vi "ConvertLVClustertoFGNetFDMString.vi"(1 "Cluster":T1={"Version"={"version"=20, "pad"=0}, "Positions"={"Doubles"={"longitude"=0.0, "latitude"=0.0, "altitude"=0.0}, "Singles"={"agl"=0.0, "phi"=0.0, "theta"=0.0, "psi"=0.0, "alpha"=0.0, "beta"=0.0}}, "Velocities"={"phidot"=0.0, "thetadot"=0.0, "psidot"=0.0, "vcas"=0.0, "climb_rate"=0.0, "v_north"=0.0, "v_east"=0.0, "v_down"=0.0, "v_wind_body_north"=0.0, "v_wind_body_east"=0.0, "v_wind_body_down"=0.0}, "Accelerations"={"A_X_pilot"=0.0, "A_Y_pilot"=0.0, "A_Z_pilot"=0.0}, "Stall"={"stall_warning"=0.0, "slip_deg"=0.0}, "Engine Status"={"num_engines"=0, "eng_state"=[0, 0, 0, 0], "rpm"=[0.0, 0.0, 0.0, 0.0], "fuel_flow"=[0.0, 0.0, 0.0, 0.0], "fuel_px"=[0.0, 0.0, 0.0, 0.0], "egt"=[0.0, 0.0, 0.0, 0.0], "cht"=[0.0, 0.0, 0.0, 0.0], "mp_osi"=[0.0, 0.0, 0.0, 0.0], "tit"=[0.0, 0.0, 0.0, 0.0], "oil_temp"=[0.0, 0.0, 0.0, 0.0], "oil_px"=[0.0, 0.0, 0.0, 0.0]}, "Consumables"={"num_tanks"=0, "fuel_quantity"=[0.0, 0.0, 0.0, 0.0]}, "Gear Status"={"num_wheels"=0, "wow"=[0, 0, 0, 0], "gear_pos"=[0.0, 0.0, 0.0, 0.0], "gear_steer"=[0.0, 0.0, 0.0, 0.0], "gear_compression"=[0.0, 0.0, 0.0, 0.0]}, "Environment"={"curr_time"=0, "warp"=0, "visibility"=0.0}, "Control Surface Positions"={"elevator"=0.0, "elevator_trim_tab"=0.0, "left_flap"=0.0, "right_flap"=0.0, "left aileron"=0.0, "right_aileron"=0.0, "rudder"=0.0, "nose_wheel"=0.0, "speedbrake"=0.0, "spoilers"=0.0}}) -> (0 "FGNetFDM":string)   [LabVIEW 2010, in "Flight Gear Interface Custom Device.lvlib"]
uses:
  Flight Gear Interface Custom Device.lvlib
  FGNetFDM.ctl
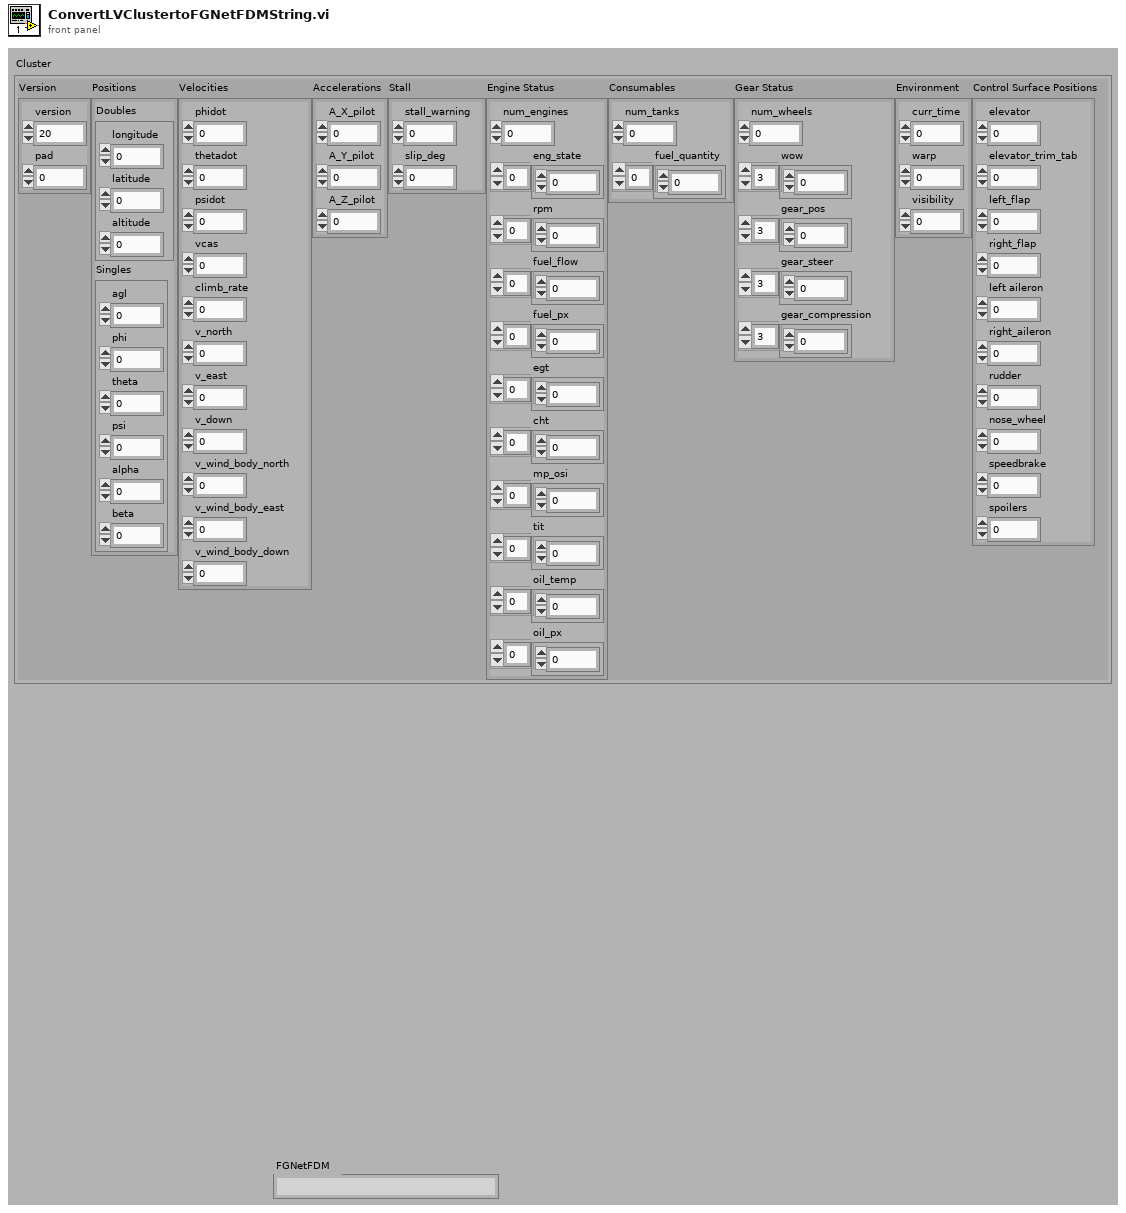
[diagram p1: front panel]
types:
  T1 = typedef "Flight Gear Interface Custom Device.lvlib/FGNetFDM.ctl" = cluster{"Version":cluster{"version":u32, "pad":u32}, "Positions":cluster{"Doubles":cluster{"longitude":dbl, "latitude":dbl, "altitude":dbl}, "Singles":cluster{"agl":sgl, "phi":sgl, "theta":sgl, "psi":sgl, "alpha":sgl, "beta":sgl}}, "Velocities":cluster{"phidot":sgl, "thetadot":sgl, "psidot":sgl, "vcas":sgl, "climb_rate":sgl, "v_north":sgl, "v_east":sgl, "v_down":sgl, "v_wind_body_north":sgl, "v_wind_body_east":sgl, "v_wind_body_down":sgl}, "Accelerations":cluster{"A_X_pilot":sgl, "A_Y_pilot":sgl, "A_Z_pilot":sgl}, "Stall":cluster{"stall_warning":sgl, "slip_deg":sgl}, "Engine Status":cluster{"num_engines":u32, "eng_state":u32[], "rpm":sgl[], "fuel_flow":sgl[], "fuel_px":sgl[], "egt":sgl[], "cht":sgl[], "mp_osi":sgl[], "tit":sgl[], "oil_temp":sgl[], "oil_px":sgl[]}, "Consumables":cluster{"num_tanks":u32, "fuel_quantity":sgl[]}, "Gear Status":cluster{"num_wheels":u32, "wow":u32[], "gear_pos":sgl[], "gear_steer":sgl[], "gear_compression":sgl[]}, "Environment":cluster{"curr_time":u32, "warp":i32, "visibility":sgl}, "Control Surface Positions":cluster{"elevator":sgl, "elevator_trim_tab":sgl, "left_flap":sgl, "right_flap":sgl, "left aileron":sgl, "right_aileron":sgl, "rudder":sgl, "nose_wheel":sgl, "speedbrake":sgl, "spoilers":sgl}}
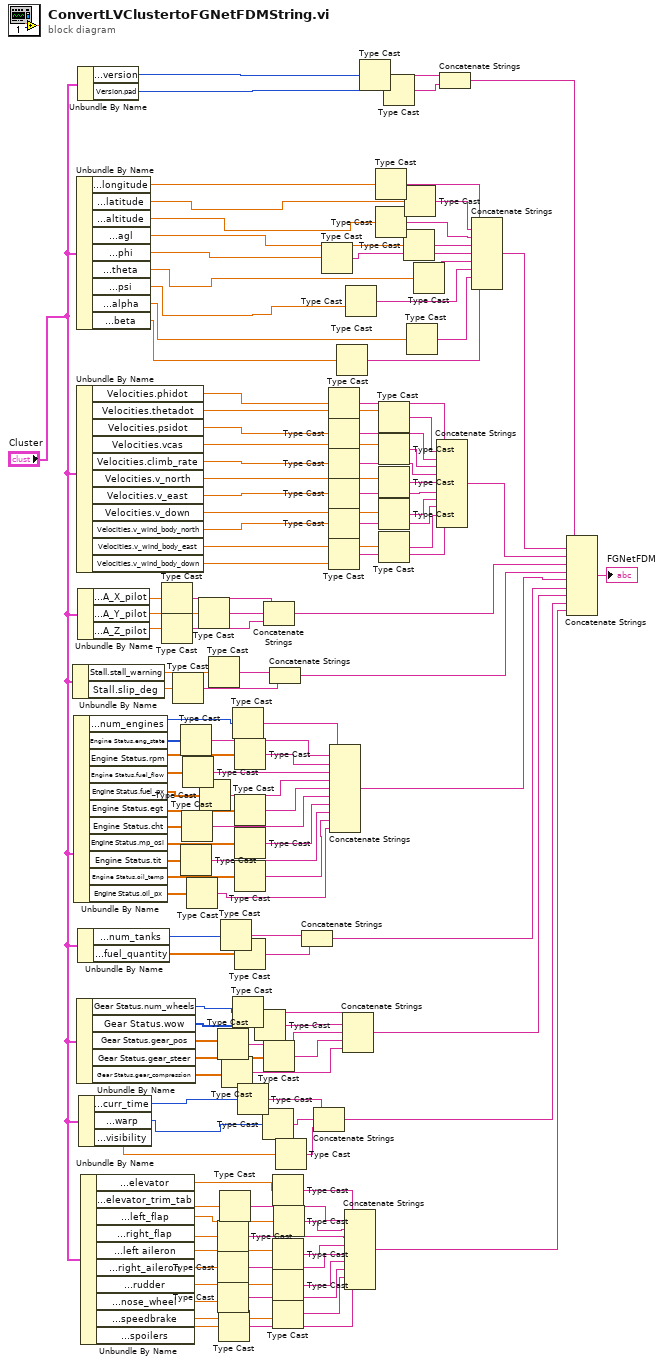
[diagram p0: block diagram]
diagram:
  n1 = Unbundle By Name("Cluster") -> ("Stall.stall_warning"=w100:sgl, "Stall.slip_deg"=w99:sgl)
  n2 = Unbundle By Name("Cluster") -> ("Engine Status.num_engines"=w7:u32, "Engine Status.eng_state"=w98:u32[], "Engine Status.rpm"=w97:sgl[], "Engine Status.fuel_flow"=w56:sgl[], "Engine Status.fuel_px"=w1:sgl[], "Engine Status.egt"=w96:sgl[], "Engine Status.cht"=w95:sgl[], "Engine Status.mp_osi"=w94:sgl[], "Engine Status.tit"=w93:sgl[], "Engine Status.oil_temp"=w92:sgl[], "Engine Status.oil_px"=w91:sgl[])
  n3 = Unbundle By Name("Cluster") -> ("Positions.Doubles.longitude"=w13:dbl, "Positions.Doubles.latitude"=w12:dbl, "Positions.Doubles.altitude"=w11:dbl, "Positions.Singles.agl"=w117:sgl, "Positions.Singles.phi"=w10:sgl, "Positions.Singles.theta"=w9:sgl, "Positions.Singles.psi"=w8:sgl, "Positions.Singles.alpha"=w116:sgl, "Positions.Singles.beta"=w115:sgl)
  n4 = Unbundle By Name("Cluster") -> ("Velocities.phidot"=w114:sgl, "Velocities.thetadot"=w108:sgl, "Velocities.psidot"=w113:sgl, "Velocities.vcas"=w107:sgl, "Velocities.climb_rate"=w112:sgl, "Velocities.v_north"=w106:sgl, "Velocities.v_east"=w111:sgl, "Velocities.v_down"=w105:sgl, "Velocities.v_wind_body_north"=w110:sgl, "Velocities.v_wind_body_east"=w104:sgl, "Velocities.v_wind_body_down"=w109:sgl)
  n5 = Unbundle By Name("Cluster") -> ("Gear Status.num_wheels"=w5:u32, "Gear Status.wow"=w89:u32[], "Gear Status.gear_pos"=w88:sgl[], "Gear Status.gear_steer"=w87:sgl[], "Gear Status.gear_compression"=w86:sgl[])
  n6 = Unbundle By Name("Cluster") -> ("Version.version"=w16:u32, "Version.pad"=w128:u32)
  n7 = Unbundle By Name("Cluster") -> ("Accelerations.A_X_pilot"=w103:sgl, "Accelerations.A_Y_pilot"=w102:sgl, "Accelerations.A_Z_pilot"=w101:sgl)
  n8 = Unbundle By Name("Cluster") -> ("Consumables.num_tanks"=w6:u32, "Consumables.fuel_quantity"=w90:sgl[])
  n9 = Unbundle By Name("Cluster") -> ("Environment.curr_time"=w15:u32, "Environment.warp"=w14:i32, "Environment.visibility"=w17:sgl)
  n10 = Unbundle By Name("Cluster") -> ("Control Surface Positions.elevator"=w85:sgl, "Control Surface Positions.elevator_trim_tab"=w84:sgl, "Control Surface Positions.left_flap"=w83:sgl, "Control Surface Positions.right_flap"=w82:sgl, "Control Surface Positions.left aileron"=w81:sgl, "Control Surface Positions.right_aileron"=w80:sgl, "Control Surface Positions.rudder"=w79:sgl, "Control Surface Positions.nose_wheel"=w78:sgl, "Control Surface Positions.speedbrake"=w77:sgl, "Control Surface Positions.spoilers"=w76:sgl)
  n11 = Type Cast(x=w103) -> (*(type *) &x=w64:string)  [unwired: 1 in]
  n12 = Type Cast(x=w101) -> (*(type *) &x=w62:string)  [unwired: 1 in]
  n13 = Type Cast(x=w99) -> (*(type *) &x=w60:string)  [unwired: 1 in]
  n14 = Type Cast(x=w98) -> (*(type *) &x=w58:string)  [unwired: 1 in]
  n15 = Type Cast(x=w93) -> (*(type *) &x=w52:string)  [unwired: 1 in]
  n16 = Type Cast(x=w95) -> (*(type *) &x=w54:string)  [unwired: 1 in]
  n17 = Type Cast(x=w56) -> (*(type *) &x=w55:string)  [unwired: 1 in]
  n18 = Type Cast(x=w91) -> (*(type *) &x=w50:string)  [unwired: 1 in]
  n19 = Type Cast(x=w102) -> (*(type *) &x=w63:string)  [unwired: 1 in]
  n20 = Type Cast(x=w1) -> (*(type *) &x=w2:string)  [unwired: 1 in]
  n21 = Type Cast(x=w100) -> (*(type *) &x=w61:string)  [unwired: 1 in]
  n22 = Type Cast(x=w88) -> (*(type *) &x=w19:string)  [unwired: 1 in]
  n23 = Type Cast(x=w82) -> (*(type *) &x=w37:string)  [unwired: 1 in]
  n24 = Type Cast(x=w80) -> (*(type *) &x=w35:string)  [unwired: 1 in]
  n25 = Type Cast(x=w78) -> (*(type *) &x=w33:string)  [unwired: 1 in]
  n26 = Type Cast(x=w76) -> (*(type *) &x=w31:string)  [unwired: 1 in]
  n27 = Type Cast(x=w84) -> (*(type *) &x=w39:string)  [unwired: 1 in]
  n28 = Type Cast(x=w6) -> (*(type *) &x=w49:string)  [unwired: 1 in]
  n29 = Type Cast(x=w86) -> (*(type *) &x=w44:string)  [unwired: 1 in]
  n30 = Type Cast(x=w7) -> (*(type *) &x=w59:string)  [unwired: 1 in]
  n31 = Type Cast(x=w5) -> (*(type *) &x=w47:string)  [unwired: 1 in]
  n32 = Type Cast(x=w97) -> (*(type *) &x=w57:string)  [unwired: 1 in]
  n33 = Type Cast(x=w96) -> (*(type *) &x=w3:string)  [unwired: 1 in]
  n34 = Type Cast(x=w94) -> (*(type *) &x=w53:string)  [unwired: 1 in]
  n35 = Type Cast(x=w92) -> (*(type *) &x=w51:string)  [unwired: 1 in]
  n36 = Type Cast(x=w90) -> (*(type *) &x=w48:string)  [unwired: 1 in]
  n37 = Type Cast(x=w15) -> (*(type *) &x=w43:string)  [unwired: 1 in]
  n38 = Type Cast(x=w89) -> (*(type *) &x=w46:string)  [unwired: 1 in]
  n39 = Type Cast(x=w14) -> (*(type *) &x=w42:string)  [unwired: 1 in]
  n40 = Concatenate Strings(w64, w63, w62) -> (w27:string)
  n41 = Type Cast(x=w87) -> (*(type *) &x=w45:string)  [unwired: 1 in]
  n42 = Concatenate Strings(w61, w60) -> (w26:string)
  n43 = Type Cast(x=w85) -> (*(type *) &x=w40:string)  [unwired: 1 in]
  n44 = Type Cast(x=w81) -> (*(type *) &x=w36:string)  [unwired: 1 in]
  n45 = Type Cast(x=w79) -> (*(type *) &x=w34:string)  [unwired: 1 in]
  n46 = Type Cast(x=w77) -> (*(type *) &x=w32:string)  [unwired: 1 in]
  n47 = Type Cast(x=w83) -> (*(type *) &x=w38:string)  [unwired: 1 in]
  n48 = Type Cast(x=w17) -> (*(type *) &x=w41:string)  [unwired: 1 in]
  n49 = Concatenate Strings(w49, w48) -> (w24:string)
  n50 = Concatenate Strings(w43, w42, w41) -> (w22:string)
  n51 = Type Cast(x=w10) -> (*(type *) &x=w122:string)  [unwired: 1 in]
  n52 = Type Cast(x=w114) -> (*(type *) &x=w75:string)  [unwired: 1 in]
  n53 = Type Cast(x=w113) -> (*(type *) &x=w73:string)  [unwired: 1 in]
  n54 = Type Cast(x=w112) -> (*(type *) &x=w71:string)  [unwired: 1 in]
  n55 = Type Cast(x=w111) -> (*(type *) &x=w69:string)  [unwired: 1 in]
  n56 = Type Cast(x=w110) -> (*(type *) &x=w67:string)  [unwired: 1 in]
  n57 = Type Cast(x=w109) -> (*(type *) &x=w65:string)  [unwired: 1 in]
  n58 = Concatenate Strings(w59, w58, w57, w55, w2, w3, w54, w53, w52, w51, w50) -> (w25:string)
  n59 = Type Cast(x=w115) -> (*(type *) &x=w118:string)  [unwired: 1 in]
  n60 = Concatenate Strings(w47, w46, w19, w45, w44) -> (w23:string)
  n61 = Concatenate Strings(w40, w39, w38, w37, w36, w35, w34, w33, w32, w31) -> (w21:string)
  n62 = Type Cast(x=w8) -> (*(type *) &x=w120:string)  [unwired: 1 in]
  n63 = Type Cast(x=w16) -> (*(type *) &x=w18:string)  [unwired: 1 in]
  n64 = Type Cast(x=w13) -> (*(type *) &x=w126:string)  [unwired: 1 in]
  n65 = Type Cast(x=w11) -> (*(type *) &x=w124:string)  [unwired: 1 in]
  n66 = Type Cast(x=w108) -> (*(type *) &x=w74:string)  [unwired: 1 in]
  n67 = Type Cast(x=w107) -> (*(type *) &x=w72:string)  [unwired: 1 in]
  n68 = Type Cast(x=w106) -> (*(type *) &x=w70:string)  [unwired: 1 in]
  n69 = Type Cast(x=w105) -> (*(type *) &x=w68:string)  [unwired: 1 in]
  n70 = Type Cast(x=w104) -> (*(type *) &x=w66:string)  [unwired: 1 in]
  n71 = Type Cast(x=w128) -> (*(type *) &x=w127:string)  [unwired: 1 in]
  n72 = Type Cast(x=w117) -> (*(type *) &x=w123:string)  [unwired: 1 in]
  n73 = Type Cast(x=w12) -> (*(type *) &x=w125:string)  [unwired: 1 in]
  n74 = Type Cast(x=w116) -> (*(type *) &x=w119:string)  [unwired: 1 in]
  n75 = Type Cast(x=w9) -> (*(type *) &x=w121:string)  [unwired: 1 in]
  n76 = Concatenate Strings(w75, w74, w73, w72, w71, w70, w69, w68, w67, w66, w65) -> (w28:string)
  n77 = Concatenate Strings(w18, w127) -> (w30:string)
  n78 = Concatenate Strings(w126, w125, w124, w123, w122, w121, w120, w119, w118) -> (w29:string)
  n79 = Concatenate Strings(w30, w29, w28, w27, w26, w25, w24, w23, w22, w21) -> (→"FGNetFDM":string)
